vi "ConfigureFrequency.vi"(8 "error in (no error)":errorcluster, 11 "Keysight44xx in":refnum<class "Keysight44xx.lvclass">) -> (0 "error out":errorcluster, 3 "Keysight44xx out":refnum<class "Keysight44xx.lvclass">)   [LabVIEW 2018, in "SpecAnPlugins.lvlib" / "Keysight44xx.lvclass"]
doc: "This function configures the frequency range, center frequency, and frequency offset. If the frequency range is equal to zero then the spectrum analyzer operates in the time-domain mode."
uses:
  Keysight44xx.lvclass
  C:/Users/ico/Documents/Projects/NistPluggableModules/SpecAn/SpecAnPlugins/SpecAnBaseClass/SpecAnBase.lvclass
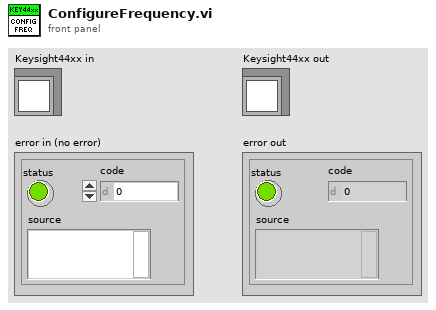
[diagram p1: front panel]
types:
  T1 = typedef "SpecAnPlugins.lvlib/SpecAnBase.lvclass/Acquisition.ctl" = cluster{"Handle":string, "Connected":bool, "Enabled":bool, "SweepModeContinuous":bool, "NumberOfSweeps":i32, "DetectorTypeAuto":bool, "DetectorType":i32, "VerticalScale":i32, "MaximumTime(seconds)":dbl}
  T2 = typedef "SpecAnPlugins.lvlib/SpecAnBase.lvclass/Frequency.ctl" = cluster{"FrequencyStart":dbl, "FrequencyStop":dbl, "FrequencyOffset":dbl}
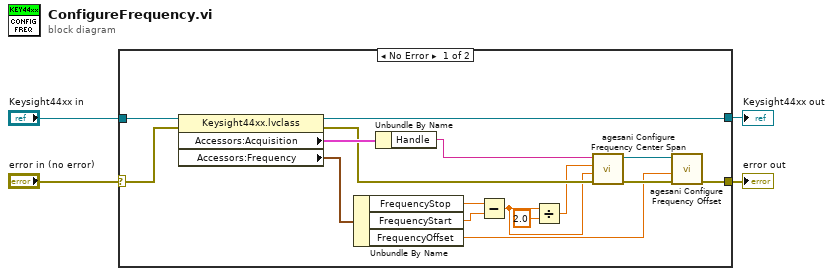
[diagram p0: block diagram]
diagram:
  n1 = case shown="No Error" "error in (no error)" {
    selector: "error in (no error)" -> [w18 w22]
    tunnel: [w13 w22] -> w3
    tunnel: "Keysight44xx in" -> [w20 w21]
    tunnel: [w19 w21] -> w1
    frame No Error {
      n2 = property class="Keysight44xx.lvclass"(reference=w20, error in=w18) -> (reference out=w19:refnum<class "Keysight44xx.lvclass">, error out=w10:errorcluster, "Accessors:Acquisition"=w16:T1, "Accessors:Frequency"=w17:T2)
      n3 = Unbundle By Name(w17) -> ("FrequencyStop"=w9:dbl, "FrequencyStart"=w8:dbl, "FrequencyOffset"=w11:dbl)
      n4 = Unbundle By Name(w16) -> ("Handle"=w15:string)
      n5 = Subtract(x=w9, y=w8) -> (x-y=w6:dbl)
      n6 = Divide(x=w6, y=2.0) -> (x/y=w5:dbl)
      n7 = call <instrlib>:"agesani Configure Frequency Center Span.vi"("error in (no error)"=w10, "span"=w6, "center frequency"=w5, "instrument handle"=w15) -> ("error out"=w12:errorcluster, "instrument handle out"=w14:refnum<k15>)  [unwired: 6 out]
      n8 = call <instrlib>:"agesani Configure Frequency Offset.vi"("error in (no error)"=w12, "frequency offset"=w11, "instrument handle"=w14) -> ("error out"=w13:errorcluster)  [unwired: 8 out]
    }
    frame Error {
    }
  }
  "error out" <- w3
  "Keysight44xx out" <- w1
